vi "Switch_Close.vi"(11 "Semiconductor Module Context":T1) -> (0 "error out":errorcluster)   [LabVIEW 2014]
uses:
  <vilib>/NI_TestStand_SemiconductorModule/NI_TestStand_Semiconductor_Module.lvlibp/PinMap/General/SemiconductorModuleContext.ctl
  <vilib>/NI_TestStand_SemiconductorModule/NI_TestStand_Semiconductor_Module.lvlibp
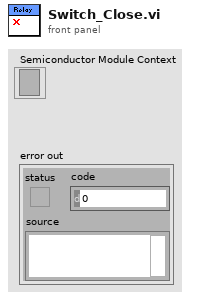
[diagram p1: front panel]
types:
  T1 = typedef "NI_TestStand_Semiconductor_Module.lvlibp/SemiconductorModuleContext.ctl" = refnum<k7>
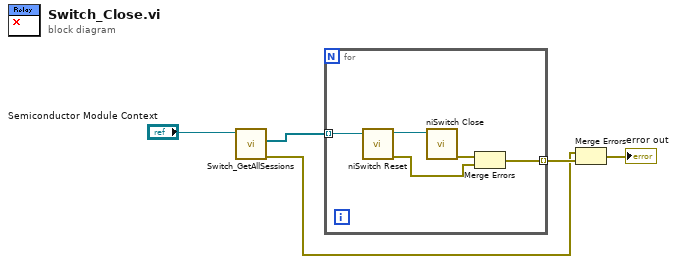
[diagram p0: block diagram]
diagram:
  n1 = call "Switch_GetAllSessions.vi"("Semiconductor Module Context"="Semiconductor Module Context") -> ("error out"=w1:errorcluster, "Instrument Sessions Data"=w4:refnum<k15>[])  [unwired: 8 in, 1 out]
  n2 = for {
    tunnel: w4 -> [w9] mode=indexing
    tunnel: [w7] -> w2 mode=indexing
    n3 = call <instrlib>:"niSwitch Reset.vi"("instrument handle"=w9) -> ("error out"=w6:errorcluster, "instrument handle out"=w8:refnum<k15>)  [unwired: 9 in]
    n4 = call <instrlib>:"niSwitch Close.vi"("instrument handle"=w8) -> ("error out"=w10:errorcluster)  [unwired: 10 in]
    n5 = Merge Errors(w10, w6) -> (w7:errorcluster)
  }
  n6 = Merge Errors(w1, w2) -> (→"error out":errorcluster)
